vi "Update Binaries.vi"() -> ()   [LabVIEW 2017]
panel:
  out "Copied dll Files":string
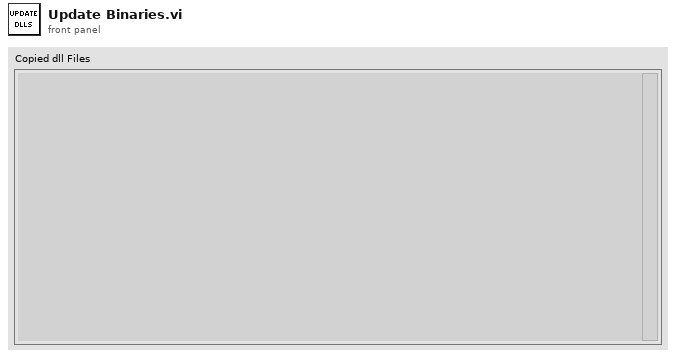
[diagram p1: front panel]
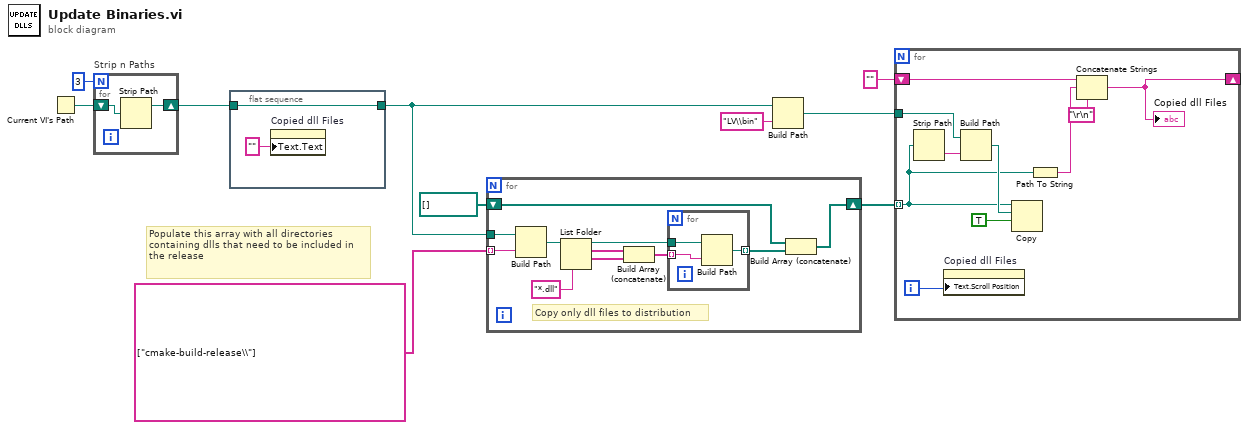
[diagram p0: block diagram]
diagram:
  # "Populate this array with all directories containing dlls that need to be included in the release"
  n1 = Current VI's Path() -> (path=w10:path)
  n2 = for "Strip n Paths" {
    N: 3 -> [_]
    shift-right: [w11] -> w3
    shift-left: w10 -> [w12]
    n3 = Strip Path(path=w12) -> (stripped path=w11:path)  [unwired: 1 out]
  }
  n4 = flat-sequence {
    tunnel: w3 -> [w14]
    tunnel: [w14] -> w2
    frame #0 {
      n5 = property on="Copied dll Files" class="Str"("Text.Text"="") -> ()  [unwired: 2 in, 2 out]
    }
  }
  n6 = for {
    tunnel: w2 -> [w19]
    tunnel: string[] ["cmake-build-release\\"] -> [w18] mode=indexing
    shift-right: [w17] -> w4
    shift-left: path[] [] -> [w16]
    # "Copy only dll files to distribution"
    n7 = Build Path(base path=w19, name or relative path=w18) -> (appended path=w25:path)
    n8 = List Folder(path=w25, pattern="*.dll") -> (path out=w21:path, filenames=w24:string[], folder names=w23:string[])  [unwired: 2 in, 1 out]
    n9 = Build Array (concatenate)(w24, w23) -> (w22:string[])
    n10 = for {
      tunnel: w22 -> [w28] mode=indexing
      tunnel: w21 -> [w27]
      tunnel: [w26] -> w15 mode=indexing
      n11 = Build Path(base path=w27, name or relative path=w28) -> (appended path=w26:path)
    }
    n12 = Build Array (concatenate)(w16, w15) -> (w17:path[])
  }
  n13 = Build Path(base path=w2, name or relative path="LV\\bin") -> (appended path=w7:path)
  n14 = for {
    tunnel: w4 -> [w34] mode=indexing
    tunnel: w7 -> [w37]
    shift-right: [w30] -> _
    shift-left: "" -> [w33]
    i -> [w29]
    n15 = Strip Path(path=w34) -> (name=w38:string)  [unwired: 1 out]
    n16 = property on="Copied dll Files" class="Str"("Text.Scroll Position"=w29) -> ()  [unwired: 2 in, 2 out]
    n17 = Build Path(base path=w37, name or relative path=w38) -> (appended path=w36:path)
    n18 = Copy(9:TRUE ("overwrite (F)"), 10:w36, 11:w34) -> ()  [unwired: 2 in, 3 out]
    n19 = Path To String(path=w34) -> (string=w32:string)
    n20 = Concatenate Strings(w33, w32, "\r\n") -> (w30:string)
    "Copied dll Files" <- w30
  }
